vi "动态优化_Test.vi"(7 "SENSOR":T1) -> (11 "动优化态前":cluster{dbl[], dbl[]}[](graph))   [LabVIEW 2020]
uses:
  Global_Variable/Global.vi
  <vilib>/ptbypt/NI_PtbyPt.lvlib
  <userlib>/_MGI/1D Array/MGI Average/MGI Average (DBL[]).vi
panel:
  in  "initialize 2":bool caption="初始化"
  in  "initialize":bool caption="初始化"
  out "PROC_1":i32
  out "Vres_min_ccw":dbl
  out "Pccw_off(%)":dbl[](array[numeric])
  in  "S_CCw":dbl[](array[numeric])
  in  "S_Cw":dbl[](array[numeric])
  in  "P_CCw":dbl[](array[numeric])
  in  "P_Cw":dbl[](array[numeric])
  out "T2ROC1+T2ROC2+T2ROC3":i32
  out "T1ROC1+T1ROC2+T1ROC3":i32
  out "T2ROC_3":i32
  out "T1ROC_3":i32
  out "OK？":bool
  out "T2_AV(%)":dbl
  out "T1_AV(%)":dbl
  out "Pcw_off(%)":dbl[](array[numeric])
  out "Vres_FD":i32
  out "Angle out":dbl
  out "Vres_min_cw":dbl
  out "T2ROC_2":i32
  out "T1ROC_2":i32
  out "PROC":i32
  out "error out":errorcluster caption="错误输出"
  in  "error in (no error)":errorcluster caption="错误输入（无错误）"
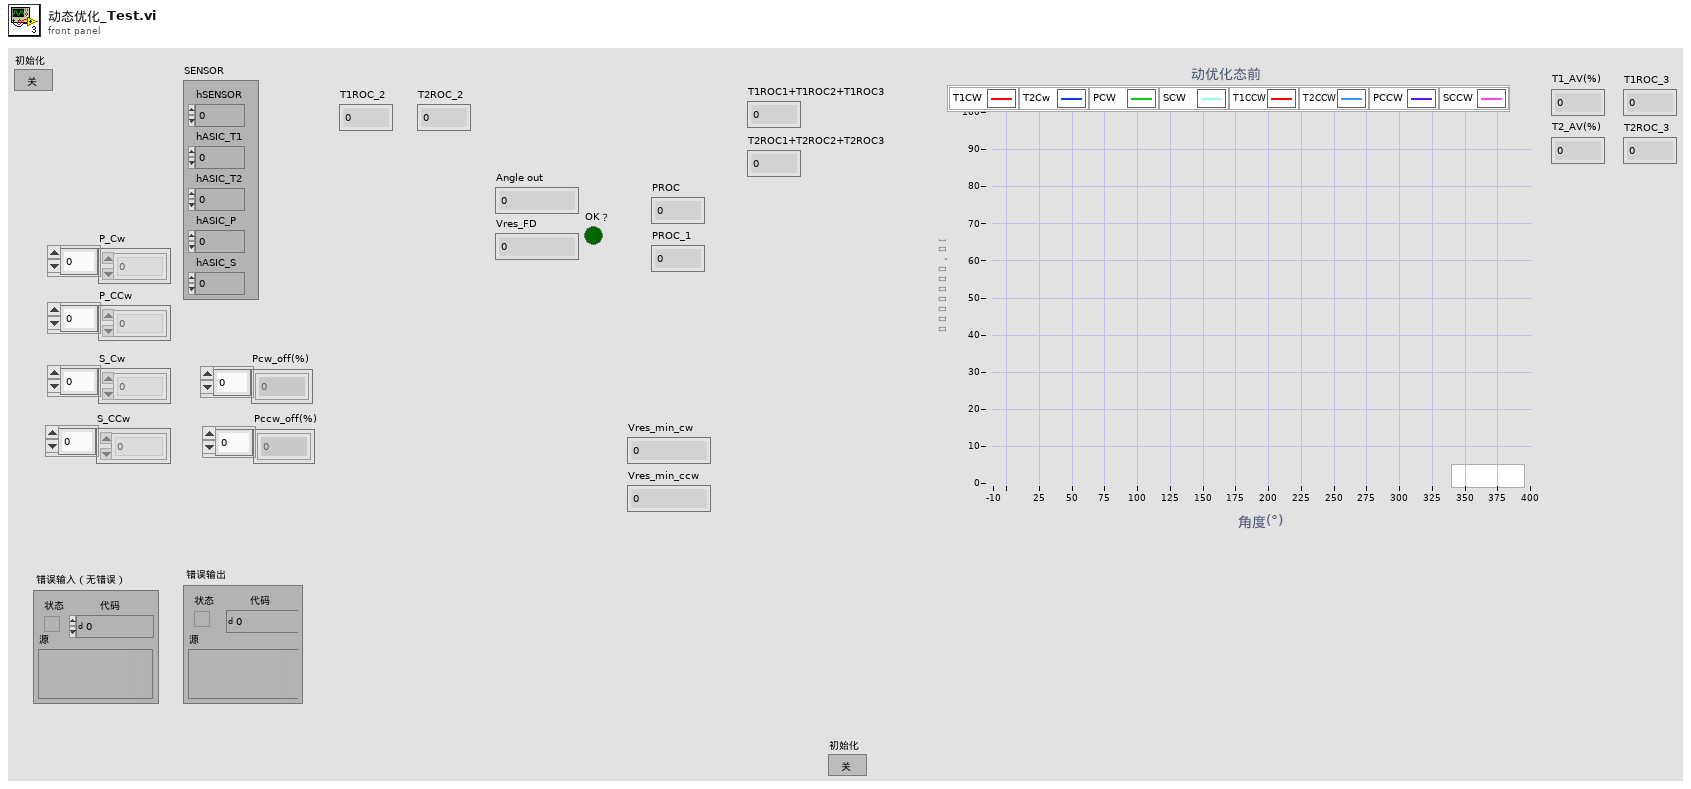
[diagram p1: front panel]
types:
  T1 = cluster{"hSENSOR":i32, "hASIC_T1":i32, "hASIC_T2":i32, "hASIC_P":i32, "hASIC_S":i32}
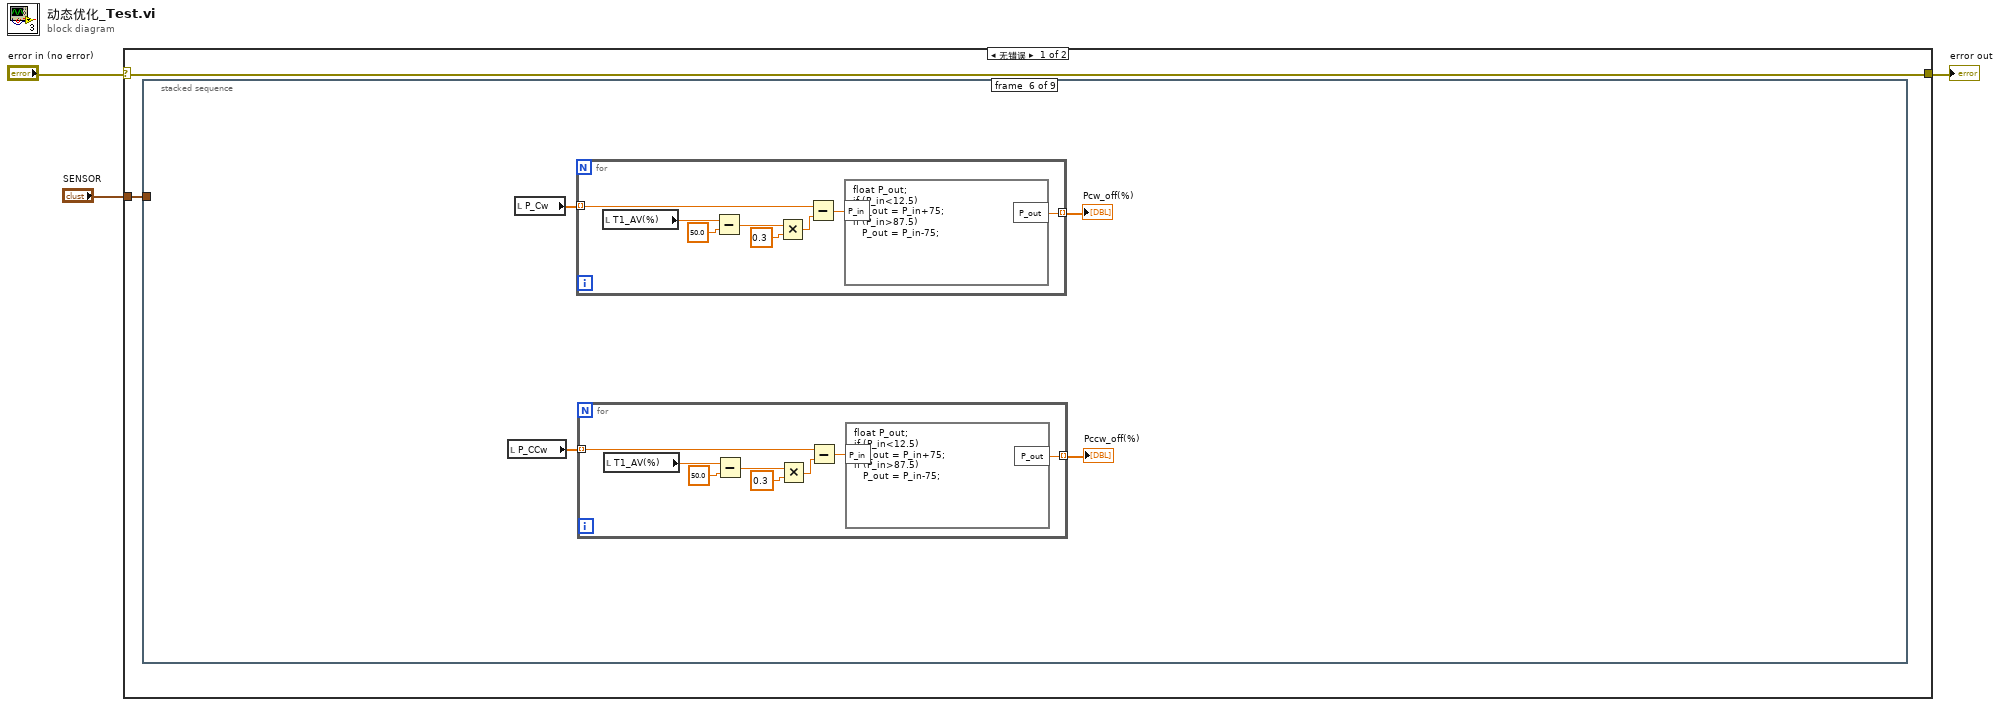
[diagram p0: block diagram]
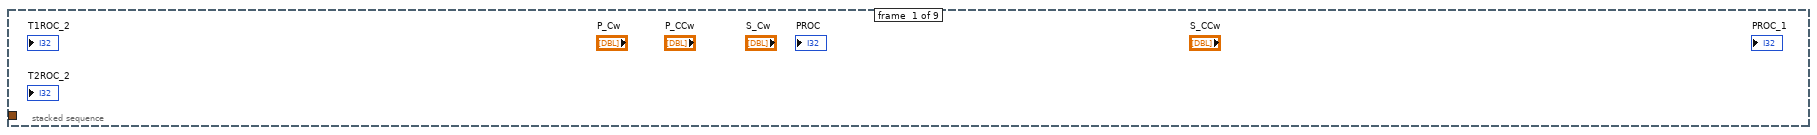
[diagram p2: hidden frame]
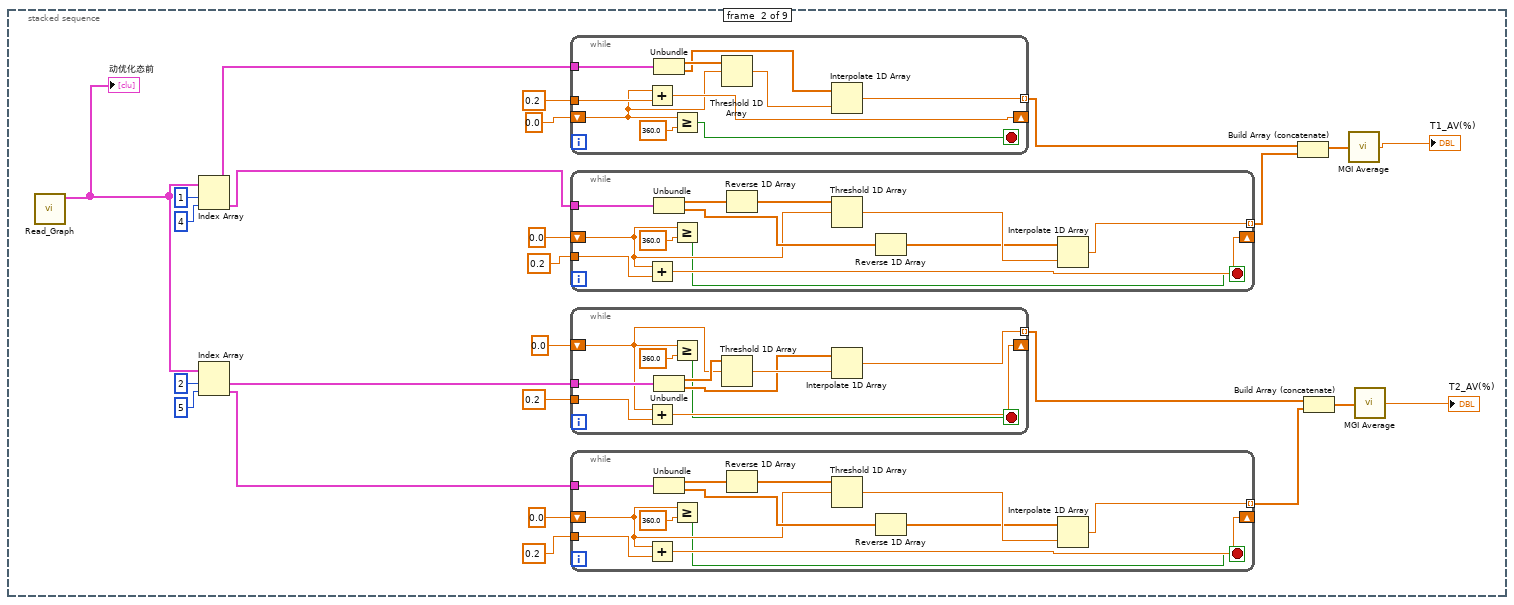
[diagram p3: hidden frame]
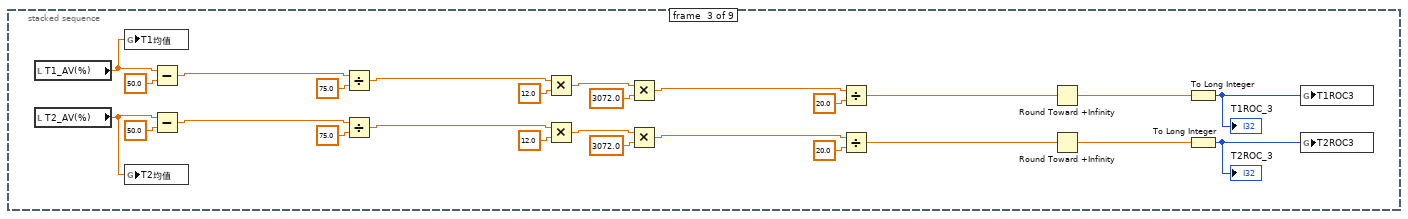
[diagram p4: hidden frame]
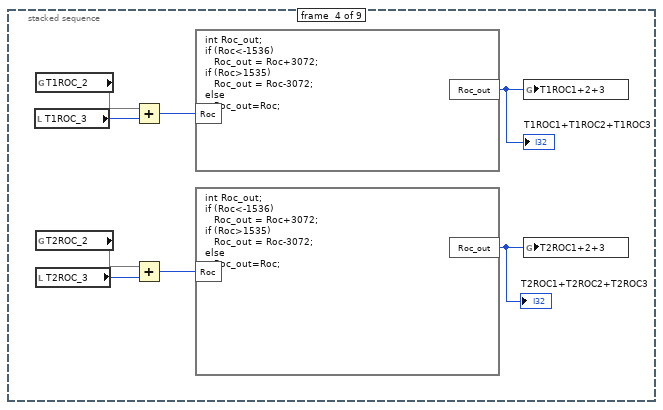
[diagram p5: hidden frame]
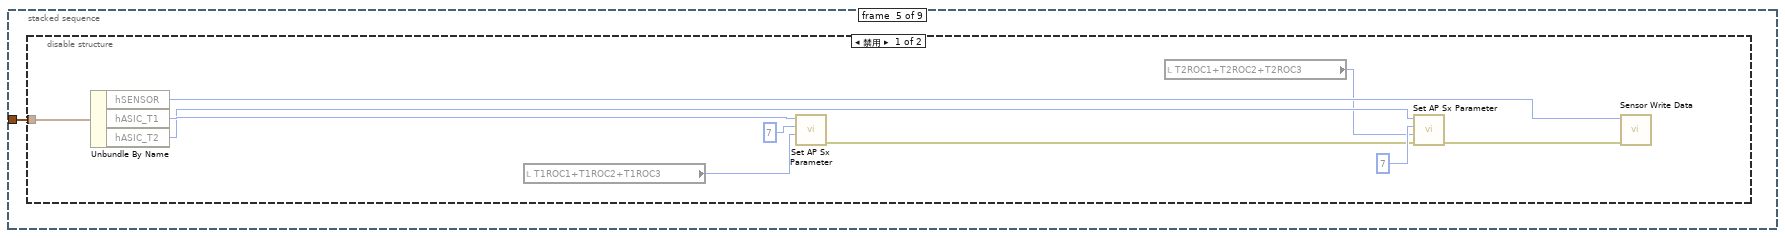
[diagram p6: hidden frame]
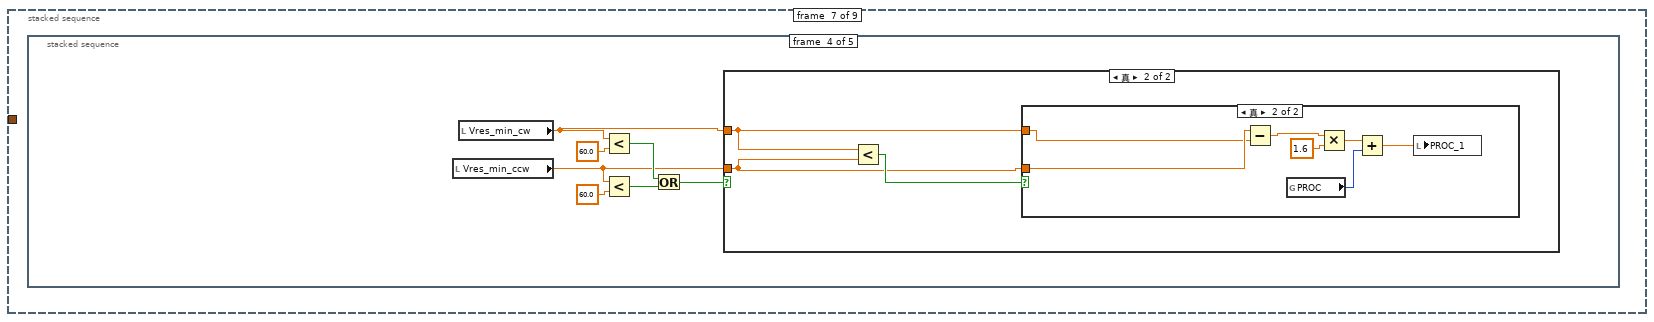
[diagram p8: hidden frame]
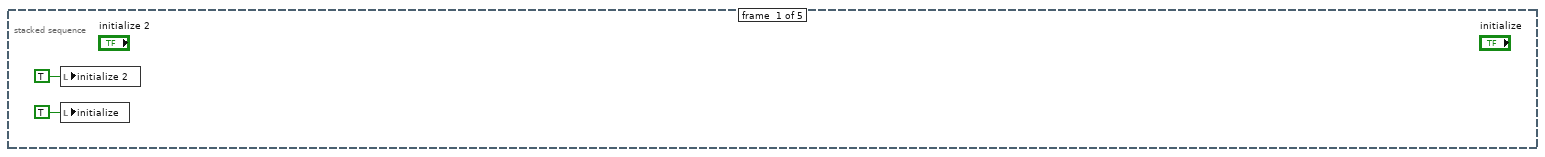
[diagram p9: hidden frame]
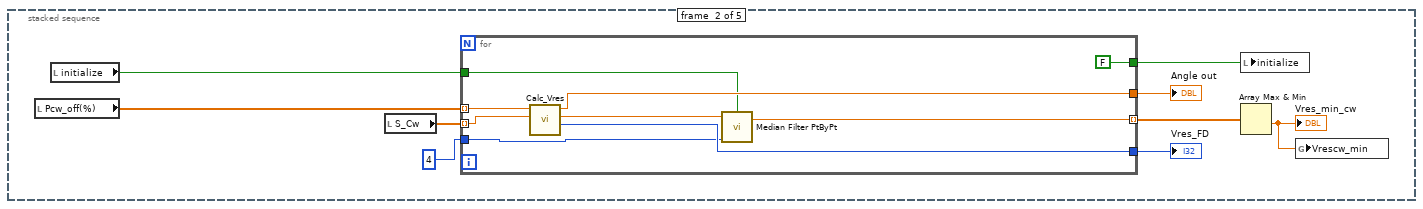
[diagram p10: hidden frame]
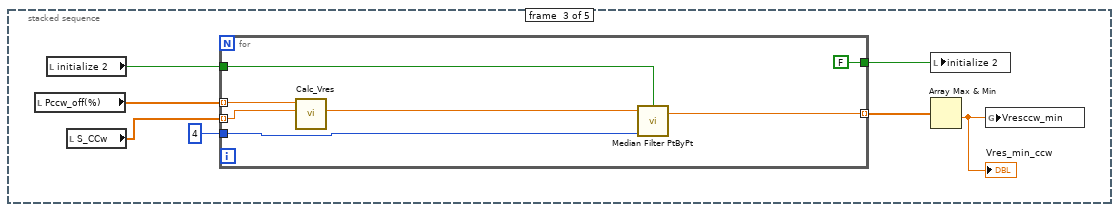
[diagram p11: hidden frame]
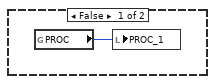
[diagram p12: hidden frame]
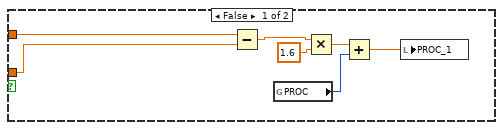
[diagram p13: hidden frame]
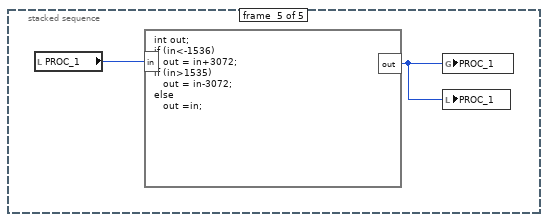
[diagram p14: hidden frame]
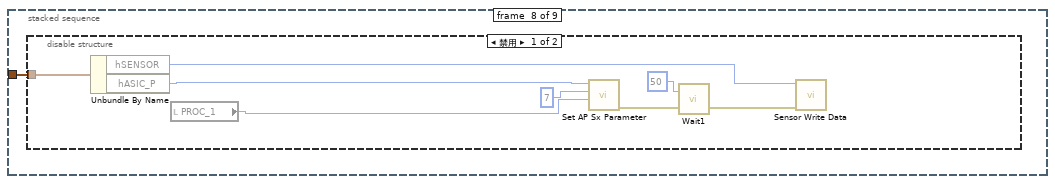
[diagram p15: hidden frame]
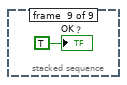
[diagram p17: hidden frame]
diagram:
  n1 = case shown="无错误" "error in (no error)" {
    selector: "error in (no error)" -> [w4 w211]
    tunnel: [w4 w211] -> w2
    tunnel: "SENSOR" -> [w5 _]
    frame No Error {
      n2 = stacked-sequence {
        tunnel: w5 -> [_ _ _ _ w109 _ _ w201 _]
        frame #0 {
        }
        frame #1 {
          n3 = call "Read_Graph.vi"() -> ("动优化态前"=w6:cluster{dbl[], dbl[]}[])  [unwired: 9 in, 2 out]
          "动优化态前" <- w6
          n4 = Index Array(array=w6, index #1=1 ("索引"), index #2=4 ("索引")) -> (element #1=w26:cluster{dbl[], dbl[]}, element #2=w21:cluster{dbl[], dbl[]})
          n5 = Index Array(array=w6, index #1=2 ("索引"), index #2=5 ("索引")) -> (element #1=w16:cluster{dbl[], dbl[]}, element #2=w15:cluster{dbl[], dbl[]})
          n6 = while {
            tunnel: w26 -> [w74]
            shift-right: [w68] -> _
            shift-left: 0.0 -> [w67]
            tunnel: [w70] -> w14 mode=indexing
            tunnel: 0.2 -> [w69]
            stop <- w65 stop-if-true
            n7 = Add(x=w67, y=w69) -> (x+y=w68:dbl)
            n8 = Unbundle(w74) -> (w73:dbl[], w71:dbl[])
            n9 = Greater Or Equal?(x=w67, y=360.0) -> (x >= y?=w65:bool)
            n10 = Threshold 1D Array(2:w67, 3:w73) -> (0:w72:dbl)  [unwired: 1 in]
            n11 = Interpolate 1D Array(1:w72, 2:w71) -> (0:w70:dbl)
          }
          n12 = while {
            tunnel: w21 -> [w64]
            shift-right: [w58] -> _
            shift-left: 0.0 -> [w57]
            tunnel: [w60] -> w13 mode=indexing
            tunnel: 0.2 -> [w59]
            stop <- w53 stop-if-true
            n13 = Add(x=w57, y=w59) -> (x+y=w58:dbl)
            n14 = Unbundle(w64) -> (w63:dbl[], w61:dbl[])
            n15 = Greater Or Equal?(x=w57, y=360.0) -> (x >= y?=w53:bool)
            n16 = Reverse 1D Array(array=w63) -> (reversed array=w55:dbl[])
            n17 = Threshold 1D Array(2:w57, 3:w55) -> (0:w62:dbl)  [unwired: 1 in]
            n18 = Reverse 1D Array(array=w61) -> (reversed array=w54:dbl[])
            n19 = Interpolate 1D Array(1:w62, 2:w54) -> (0:w60:dbl)
          }
          n20 = while {
            tunnel: w16 -> [w52]
            shift-right: [w46] -> _
            shift-left: 0.0 -> [w45]
            tunnel: [w48] -> w9 mode=indexing
            tunnel: 0.2 -> [w47]
            stop <- w43 stop-if-true
            n21 = Add(x=w45, y=w47) -> (x+y=w46:dbl)
            n22 = Unbundle(w52) -> (w51:dbl[], w49:dbl[])
            n23 = Greater Or Equal?(x=w45, y=360.0) -> (x >= y?=w43:bool)
            n24 = Threshold 1D Array(2:w45, 3:w51) -> (0:w50:dbl)  [unwired: 1 in]
            n25 = Interpolate 1D Array(1:w50, 2:w49) -> (0:w48:dbl)
          }
          n26 = while {
            tunnel: w15 -> [w42]
            shift-right: [w36] -> _
            shift-left: 0.0 -> [w35]
            tunnel: [w38] -> w12 mode=indexing
            tunnel: 0.2 -> [w37]
            stop <- w31 stop-if-true
            n27 = Add(x=w35, y=w37) -> (x+y=w36:dbl)
            n28 = Unbundle(w42) -> (w41:dbl[], w39:dbl[])
            n29 = Greater Or Equal?(x=w35, y=360.0) -> (x >= y?=w31:bool)
            n30 = Reverse 1D Array(array=w41) -> (reversed array=w32:dbl[])
            n31 = Threshold 1D Array(2:w35, 3:w32) -> (0:w40:dbl)  [unwired: 1 in]
            n32 = Reverse 1D Array(array=w39) -> (reversed array=w33:dbl[])
            n33 = Interpolate 1D Array(1:w40, 2:w33) -> (0:w38:dbl)
          }
          n34 = Build Array (concatenate)(w14, w13) -> (w11:dbl[])
          n35 = Build Array (concatenate)(w9, w12) -> (w10:dbl[])
          n36 = call-poly <userlib>:"MGI Average.vi"("Double[]"=w11) -> ("Average"=→"T1_AV(%)":dbl)  [unwired: 1 in]
          n37 = call-poly <userlib>:"MGI Average.vi"("Double[]"=w10) -> ("Average"=→"T2_AV(%)":dbl)  [unwired: 1 in]
        }
        frame #2 {
          n38 = local read "T1_AV(%)"() -> (w76:dbl)
          n39 = local read "T2_AV(%)"() -> (w75:dbl)
          n40 = global write "Global.vi" "T1均值"(w76) -> ()
          n41 = global write "Global.vi" "T2均值"(w75) -> ()
          n42 = Subtract(x=w76, y=50.0) -> (x-y=w99:dbl)
          n43 = Subtract(x=w75, y=50.0) -> (x-y=w88:dbl)
          n44 = Divide(x=w99, y=75.0) -> (x/y=w97:dbl)
          n45 = Divide(x=w88, y=75.0) -> (x/y=w90:dbl)
          n46 = Multiply(x=w97, y=12.0) -> (x*y=w84:dbl)
          n47 = Multiply(x=w90, y=12.0) -> (x*y=w85:dbl)
          n48 = Multiply(x=w84, y=3072.0) -> (x*y=w82:dbl)
          n49 = Multiply(x=w85, y=3072.0) -> (x*y=w83:dbl)
          n50 = Divide(x=w82, y=20.0) -> (x/y=w86:dbl)
          n51 = Divide(x=w83, y=20.0) -> (x/y=w81:dbl)
          n52 = Round Toward +Infinity(x=w86) -> (ceil(x): smallest int >= x=w79:dbl)
          n53 = Round Toward +Infinity(x=w81) -> (ceil(x): smallest int >= x=w80:dbl)
          n54 = To Long Integer(number=w79) -> (32bit integer=w78:i32)
          "T1ROC_3" <- w78
          n55 = To Long Integer(number=w80) -> (32bit integer=w77:i32)
          "T2ROC_3" <- w77
          n56 = global write "Global.vi" "T1ROC3"(w78) -> ()
          n57 = global write "Global.vi" "T2ROC3"(w77) -> ()
        }
        frame #3 {
          n58 = local read "T1ROC_3"() -> (w108:i32)
          n59 = global read "Global.vi" "T1ROC_2"() -> (w102)
          n60 = global read "Global.vi" "T2ROC_2"() -> (w101)
          n61 = local read "T2ROC_3"() -> (w105:i32)
          n62 = Add(x=w102, y=w108) -> (x+y=w107:i32)
          n63 = Add(x=w101, y=w105) -> (x+y=w106:i32)
          n64 = formula code="int Roc_out;\nif (Roc<-1536)\n   Roc_out = Roc+3072;\nif (Roc>1535)\n   Roc_out = Roc-3072;\nelse\n   Roc_out=Roc;"("Roc"=w107) -> ("Roc_out"=w104:i32)
          "T1ROC1+T1ROC2+T1ROC3" <- w104
          n65 = formula code="int Roc_out;\nif (Roc<-1536)\n   Roc_out = Roc+3072;\nif (Roc>1535)\n   Roc_out = Roc-3072;\nelse\n   Roc_out=Roc;"("Roc"=w106) -> ("Roc_out"=w103:i32)
          "T2ROC1+T2ROC2+T2ROC3" <- w103
          n66 = global write "Global.vi" "T1ROC1+2+3"(w104) -> ()
          n67 = global write "Global.vi" "T2ROC1+2+3"(w103) -> ()
        }
        frame #4 {
          n68 = disable-structure shown="禁用" {
            disable-tunnel: w109 -> [w119 _]
            frame Disabled {
              n69 = Unbundle By Name(w119) -> ("hSENSOR"=w116:i32, "hASIC_T1"=w118:i32, "hASIC_T2"=w117:i32)
              n70 = local read "T1ROC1+T1ROC2+T1ROC3"() -> (w111:i32)
              n71 = call "Set AP Sx Parameter.vi"("para2"=w111, "asicBitsName"=7, "asicHandle"=w118) -> ("error out"=w113:errorcluster)  [unwired: 7 in, 1 out]
              n72 = local read "T2ROC1+T2ROC2+T2ROC3"() -> (w110:i32)
              n73 = call "Set AP Sx Parameter.vi"("error in (no error)"=w113, "para2"=w110, "asicBitsName"=7, "asicHandle"=w117) -> ("error out"=w112:errorcluster)  [unwired: 6 in, 1 out]
              n74 = call "Sensor Write Data.vi"("error in (no error)"=w112, "sensorHandle"=w116) -> ()  [unwired: 8 in, 2 out]
            }
            frame Enabled {
            }
          }
        }
        frame #5 {
          n75 = local read "P_CCw"() -> (w120:dbl[])
          n76 = local read "P_Cw"() -> (w123:dbl[])
          n77 = for {
            tunnel: w123 -> [w133] mode=indexing
            tunnel: [w132] -> w122 mode=indexing
            n78 = local read "T1_AV(%)"() -> (w139:dbl)
            n79 = Subtract(x=w139, y=50.0) -> (x-y=w137:dbl)
            n80 = Multiply(x=w137, y=0.3) -> (x*y=w135:dbl)
            n81 = Subtract(x=w133, y=w135) -> (x-y=w134:dbl)
            n82 = formula code="float P_out;\nif (P_in<12.5)\n   P_out = P_in+75;\nif (P_in>87.5)\n   P_out = P_in-75;"("P_in"=w134) -> ("P_out"=w132:dbl)
          }
          "Pcw_off(%)" <- w122
          n83 = for {
            tunnel: w120 -> [w125] mode=indexing
            tunnel: [w124] -> w121 mode=indexing
            n84 = local read "T1_AV(%)"() -> (w131:dbl)
            n85 = Subtract(x=w131, y=50.0) -> (x-y=w129:dbl)
            n86 = Multiply(x=w129, y=0.3) -> (x*y=w127:dbl)
            n87 = Subtract(x=w125, y=w127) -> (x-y=w126:dbl)
            n88 = formula code="float P_out;\nif (P_in<12.5)\n   P_out = P_in+75;\nif (P_in>87.5)\n   P_out = P_in-75;"("P_in"=w126) -> ("P_out"=w124:dbl)
          }
          "Pccw_off(%)" <- w121
        }
        frame #6 {
          n89 = stacked-sequence {
            frame #0 {
              n90 = local write "initialize 2"(TRUE ("initialize 2")) -> ()
              n91 = local write "initialize"(TRUE ("initialize")) -> ()
            }
            frame #1 {
              n92 = local read "Pcw_off(%)"() -> (w149:dbl[])
              n93 = local read "initialize"() -> (w143:bool)
              n94 = local read "S_Cw"() -> (w148:dbl[])
              n95 = for {
                tunnel: [w156] -> w147
                tunnel: [w159] -> w150
                tunnel: w148 -> [w158] mode=indexing
                tunnel: [w154] -> w146 mode=indexing
                tunnel: w149 -> [w157] mode=indexing
                tunnel: 4 ("rank") -> [w153]
                tunnel: w143 -> [w152]
                tunnel: [FALSE ("initialize")] -> w142
                n96 = call "Calc_Vres.vi"("S_Data in"=w158, "P_Data in"=w157) -> ("Vres_FD"=w159:i32, "Vres"=w155:dbl, "Angle out"=w156:dbl)  [unwired: 7 in]
                n97 = call <vilib>:"Median Filter PtByPt.vi"("initialize"=w152, "rank"=w153, "x"=w155) -> ("Filtered x"=w154:dbl)  [unwired: 1 in, 1 out]
              }
              "Angle out" <- w147
              "Vres_FD" <- w150
              n98 = local write "initialize"(w142) -> ()
              n99 = Array Max & Min(array=w146) -> (min value=w145:dbl)  [unwired: 3 out]
              "Vres_min_cw" <- w145
              n100 = global write "Global.vi" "Vrescw_min"(w145) -> ()
            }
            frame #2 {
              n101 = local read "Pccw_off(%)"() -> (w166:dbl[])
              n102 = local read "initialize 2"() -> (w161:bool)
              n103 = local read "S_CCw"() -> (w165:dbl[])
              n104 = for {
                tunnel: w165 -> [w173] mode=indexing
                tunnel: [w170] -> w164 mode=indexing
                tunnel: w166 -> [w172] mode=indexing
                tunnel: 4 ("rank") -> [w169]
                tunnel: w161 -> [w168]
                tunnel: [FALSE ("initialize 2")] -> w160
                n105 = call "Calc_Vres.vi"("S_Data in"=w173, "P_Data in"=w172) -> ("Vres"=w171:dbl)  [unwired: 7 in, 2 out]
                n106 = call <vilib>:"Median Filter PtByPt.vi"("initialize"=w168, "rank"=w169, "x"=w171) -> ("Filtered x"=w170:dbl)  [unwired: 1 in, 1 out]
              }
              n107 = local write "initialize 2"(w160) -> ()
              n108 = Array Max & Min(array=w164) -> (min value=w163:dbl)  [unwired: 3 out]
              "Vres_min_ccw" <- w163
              n109 = global write "Global.vi" "Vresccw_min"(w163) -> ()
            }
            frame #3 {
              n110 = local read "Vres_min_ccw"() -> (w175:dbl)
              n111 = local read "Vres_min_cw"() -> (w176:dbl)
              n112 = Less?(x=w176, y=60.0) -> (x < y?=w178:bool)
              n113 = Less?(x=w175, y=60.0) -> (x < y?=w177:bool)
              n114 = Or(x=w178, y=w177) -> (x .or. y?=w174:bool)
              n115 = case shown="真" w174 {
                tunnel: w176 -> [_ w183]
                tunnel: w175 -> [_ w182]
                frame False {
                  n116 = global read "Global.vi" "PROC"() -> (w181:i32)
                  n117 = local write "PROC_1"(w181) -> ()
                }
                frame True {
                  n118 = Less?(x=w183, y=w182) -> (x < y?=w184:bool)
                  n119 = case shown="真" w184 {
                    tunnel: w182 -> [w189 w198]
                    tunnel: w183 -> [w190 w197]
                    frame False {
                      n120 = Subtract(x=w190, y=w189) -> (x-y=w191:dbl)
                      n121 = global read "Global.vi" "PROC"() -> (w187:i32)
                      n122 = Multiply(x=w191, y=1.6) -> (x*y=w185:dbl)
                      n123 = Add(x=w185, y=w187) -> (x+y=w186:dbl)
                      n124 = local write "PROC_1"(w186) -> ()
                    }
                    frame True {
                      n125 = Subtract(x=w198, y=w197) -> (x-y=w195:dbl)
                      n126 = global read "Global.vi" "PROC"() -> (w194:i32)
                      n127 = Multiply(x=w195, y=1.6) -> (x*y=w192:dbl)
                      n128 = Add(x=w192, y=w194) -> (x+y=w193:dbl)
                      n129 = local write "PROC_1"(w193) -> ()
                    }
                  }
                }
              }
            }
            frame #4 {
              n130 = local read "PROC_1"() -> (w200:i32)
              n131 = formula code="int out;\nif (in<-1536)\n   out = in+3072;\nif (in>1535)\n   out = in-3072;\nelse\n   out =in;"("in"=w200) -> ("out"=w199:i32)
              n132 = global write "Global.vi" "PROC_1"(w199) -> ()
              n133 = local write "PROC_1"(w199) -> ()
            }
          }
        }
        frame #7 {
          n134 = disable-structure shown="禁用" {
            disable-tunnel: w201 -> [w209 _]
            frame Disabled {
              n135 = Unbundle By Name(w209) -> ("hSENSOR"=w207:i32, "hASIC_P"=w208:i32)
              n136 = local read "PROC_1"() -> (w202:i32)
              n137 = call "Set AP Sx Parameter.vi"("para2"=w202, "asicBitsName"=7, "asicHandle"=w208) -> ("error out"=w206:errorcluster)  [unwired: 7 in, 1 out]
              n138 = call "Wait1.vi"("error in (no error)"=w206, "Wait（150ms）"=u32 50) -> ("error out"=w205:errorcluster)  [unwired: 1 in]
              n139 = call "Sensor Write Data.vi"("error in (no error)"=w205, "sensorHandle"=w207) -> ()  [unwired: 8 in, 2 out]
            }
            frame Enabled {
            }
          }
        }
        frame #8 {
          "OK？" <- TRUE ("OK？")
        }
      }
    }
    frame Error {
    }
  }
  "error out" <- w2
